vi "Status Scan.vi"(0 "VISA resource name":refnum<visa-resource-name>, 11 "error in (no error)":errorcluster) -> (4 "VISA resource name out":refnum<visa-resource-name>, 6 "Scan Channel (1)":i32=1 min=1 max=16 step=1, 8 "Autoscan":bool, 15 "error out":errorcluster)   [LabVIEW 2021, in "Lake Shore Cryotronics 370.lvlib"]
doc: "This VI indicates which channel is being scanned and if the Autoscan feature is active. Functions only when the Model 3716 Scanner is installed."
uses:
  Lake Shore Cryotronics 370.lvlib
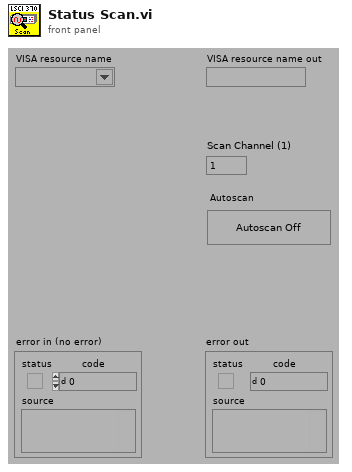
[diagram p1: front panel]
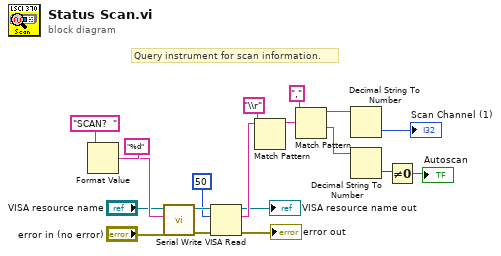
[diagram p0: block diagram]
diagram:
  # "Query instrument for scan information."
  n1 = Format Value(string ("")="SCAN?  ", format string="%d") -> (output string=w8:string)  [unwired: 1 in]
  n2 = call "Serial Write.vi"("error in (no error)"="error in (no error)", "Write Buffer (\"\")"=w8, "VISA resource name"="VISA resource name") -> ("error out"=w18:errorcluster, "VISA resource name out"=w19:refnum<visa-resource-name>)  [unwired: 6 in, 1 out]
  n3 = VISA Read(VISA resource name=w19, byte count=50, error in (no error)=w18) -> (VISA resource name out=→"VISA resource name out":refnum<visa-resource-name>, read buffer=w16:string, error out=→"error out":errorcluster)  [unwired: 1 out]
  n4 = Match Pattern(string=w16, regular expression="\\r") -> (before substring=w13:string)  [unwired: 1 in, 3 out]
  n5 = Match Pattern(string=w13, regular expression=",") -> (before substring=w12:string, after substring=w11:string)  [unwired: 1 in, 2 out]
  n6 = Decimal String To Number(string=w12) -> (number=→"Scan Channel (1)":i32)  [unwired: 2 in, 1 out]
  n7 = Decimal String To Number(string=w11) -> (number=w4:i32)  [unwired: 2 in, 1 out]
  n8 = Not Equal To 0?(x=w4) -> (x != 0?=→"Autoscan":bool)
